vi "Query Capabilities (Macro Command).vi"(0 "VISA resource name":refnum<visa-resource-name>, 5 "Absolute Maximums (T)":bool=TRUE, 11 "error in (no error)":errorcluster) -> (4 "VISA resource name out":refnum<visa-resource-name>, 6 "Number of Commands":u32 max=12 step=1, 8 "Delay Min":dbl, 10 "Delay Max":dbl, 15 "error out":errorcluster)   [LabVIEW 2020, in "NH Research Regenerative Test Series.lvlib"]
doc: "This will query the maximum number of commands and the absolute minimum and maximum legal values for the time interval for macros."
uses:
  NH Research Regenerative Test Series.lvlib
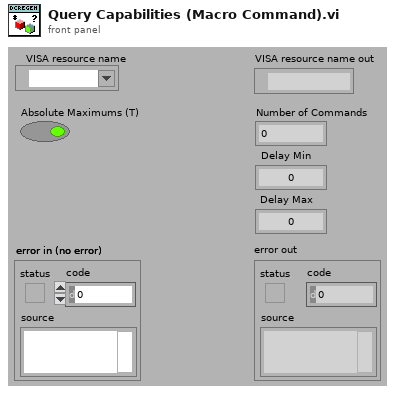
[diagram p1: front panel]
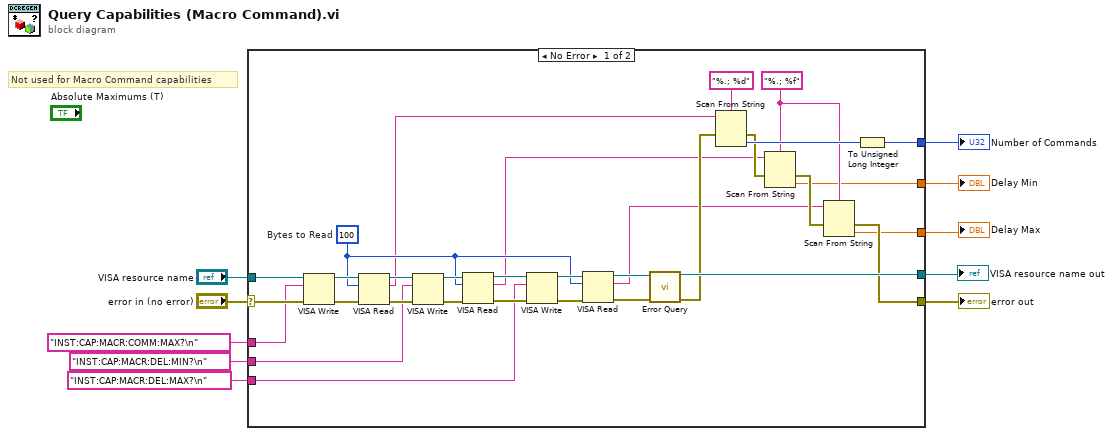
[diagram p0: block diagram]
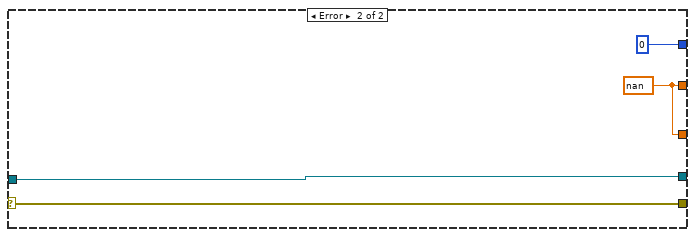
[diagram p2: hidden frame]
diagram:
  # "Not used for Macro Command capabilities"
  n1 = case shown="No Error" "error in (no error)" {
    selector: "error in (no error)" -> [w40 w46]
    tunnel: [w17 w46] -> w9
    tunnel: [w38 w45] -> w7
    tunnel: "VISA resource name" -> [w39 w45]
    tunnel: [w35 u32 0] -> w6
    tunnel: "INST:CAP:MACR:COMM:MAX?\n" ("write buffer") -> [w28 _]
    tunnel: "INST:CAP:MACR:DEL:MIN?\n" ("write buffer") -> [w27 _]
    tunnel: "INST:CAP:MACR:DEL:MAX?\n" ("write buffer") -> [w26 _]
    tunnel: [w15 w43] -> w2
    tunnel: [w14 w43] -> w1
    frame No Error {
      w16 = "%.; %f" ("format string")
      w23 = u32 100  # Bytes to Read
      n2 = VISA Write(VISA resource name=w39, write buffer=w28, error in (no error)=w40) -> (VISA resource name out=w41:refnum<visa-resource-name>, error out=w42:errorcluster)  [unwired: 1 out]
      n3 = VISA Read(VISA resource name=w41, byte count=w23, error in (no error)=w42) -> (VISA resource name out=w25:refnum<visa-resource-name>, read buffer=w13:string, error out=w30:errorcluster)  [unwired: 1 out]
      n4 = VISA Write(VISA resource name=w25, write buffer=w27, error in (no error)=w30) -> (VISA resource name out=w33:refnum<visa-resource-name>, error out=w34:errorcluster)  [unwired: 1 out]
      n5 = VISA Read(VISA resource name=w33, byte count=w23, error in (no error)=w34) -> (VISA resource name out=w24:refnum<visa-resource-name>, read buffer=w12:string, error out=w29:errorcluster)  [unwired: 1 out]
      n6 = VISA Write(VISA resource name=w24, write buffer=w26, error in (no error)=w29) -> (VISA resource name out=w31:refnum<visa-resource-name>, error out=w32:errorcluster)  [unwired: 1 out]
      n7 = VISA Read(VISA resource name=w31, byte count=w23, error in (no error)=w32) -> (VISA resource name out=w21:refnum<visa-resource-name>, read buffer=w11:string, error out=w22:errorcluster)  [unwired: 1 out]
      n8 = call "Error Query.vi"("VISA resource name"=w21, "error in (no error)"=w22) -> ("VISA resource name out"=w38:refnum<visa-resource-name>, "error out"=w37:errorcluster)  [unwired: 10 in, 2 out]
      n9 = Scan From String(format string="%.; %d", input string=w13, error in=w37) -> (error out=w19:errorcluster, output 1=w36:i32)  [unwired: 2 in, 2 out]
      n10 = Scan From String(format string=w16, input string=w12, error in=w19) -> (error out=w18:errorcluster, output 1=w15:dbl)  [unwired: 2 in, 2 out]
      n11 = Scan From String(format string=w16, input string=w11, error in=w18) -> (error out=w17:errorcluster, output 1=w14:dbl)  [unwired: 2 in, 2 out]
      n12 = To Unsigned Long Integer(number=w36) -> (unsigned 32bit integer=w35:u32)
    }
    frame Error {
      w43 = nan
    }
  }
  "error out" <- w9
  "VISA resource name out" <- w7
  "Number of Commands" <- w6
  "Delay Min" <- w2
  "Delay Max" <- w1
